vi "task.vi"() -> ()   [LabVIEW 2016, in "DGUS.lvlib"]
uses:
  DGUS.lvlib
  Control/state.ctl
  Control/data.ctl
  DGUS.lvclass
  <vilib>/Instr/_visa.llb/VISA Configure Serial Port (Instr).vi
panel:
  in  "停止":bool
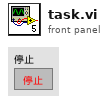
[diagram p1: front panel]
types:
  T1 = typedef "DGUS.lvlib/state.ctl" = enum16{"init", "open", "get data", "write buffer", "read buffer", "exit"}
  T2 = typedef "DGUS.lvlib/data.ctl" = cluster{"DGUS.lvclass":refnum<class "DGUS.lvclass">, "msgQueen":refnum<queue>, "VISA resource name":refnum<visa-resource-name>, "WriteBuffer":string, "ReadBuffer":string}
  T3 = cluster{"站点名称":string, "中文名称":string, "英文名称":string, "检测值":sgl, "小数位":u8, "单位":string, "页面":u16}[]
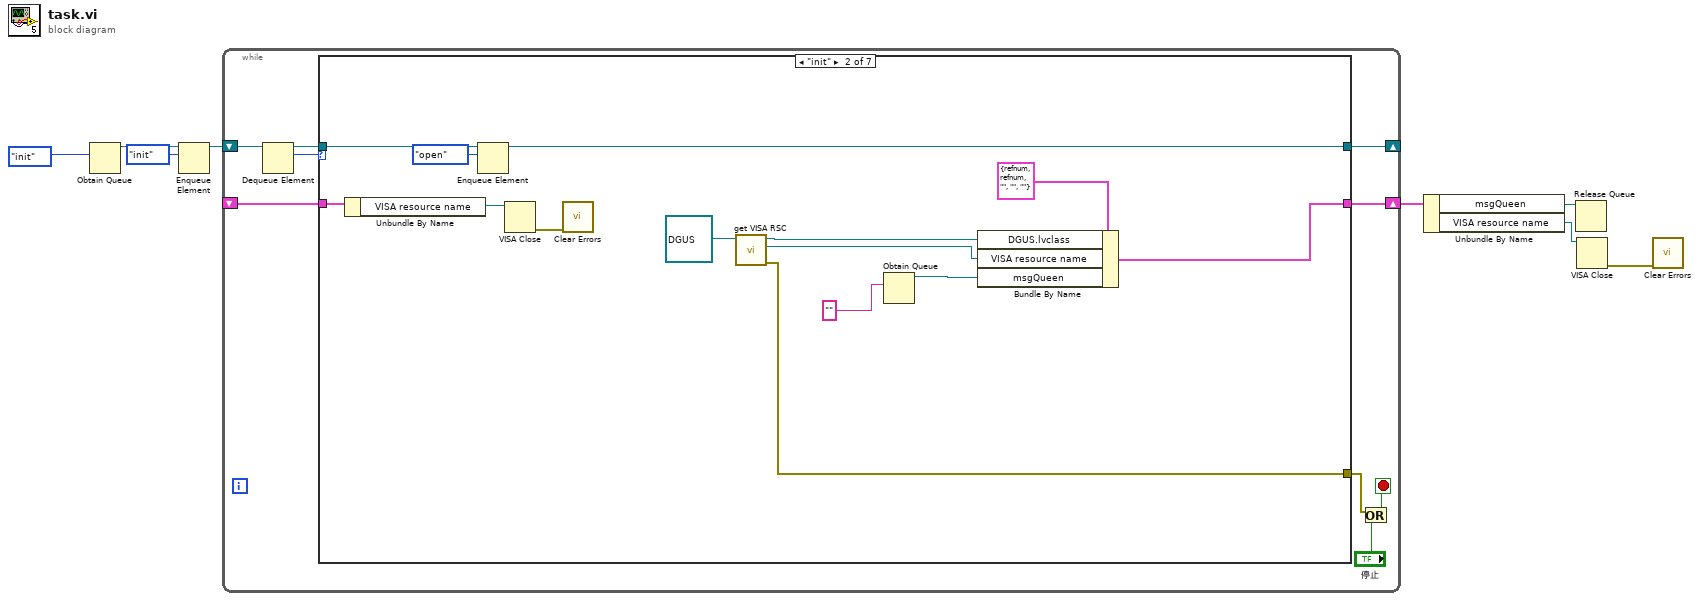
[diagram p0: block diagram]
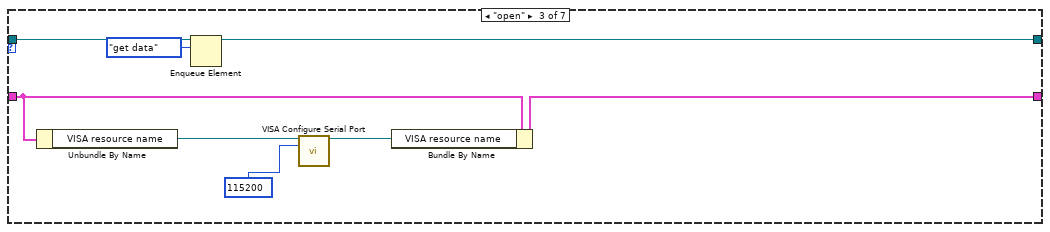
[diagram p3: hidden frame]
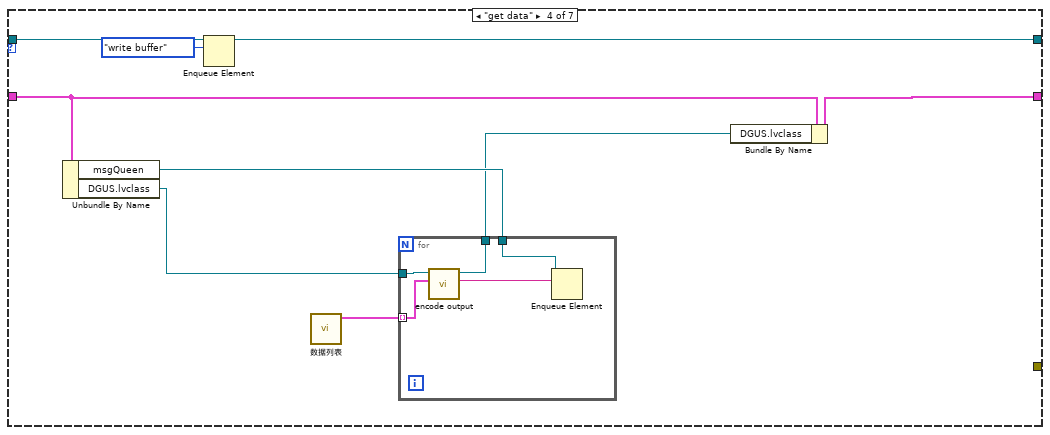
[diagram p4: hidden frame]
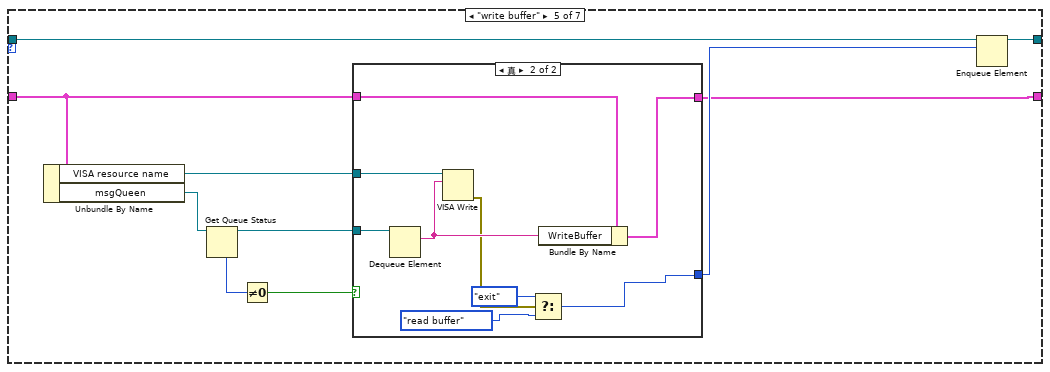
[diagram p5: hidden frame]
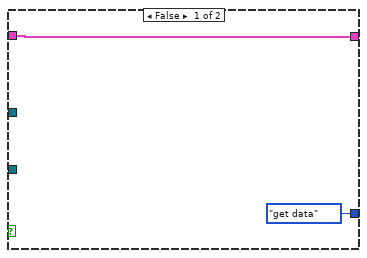
[diagram p6: hidden frame]
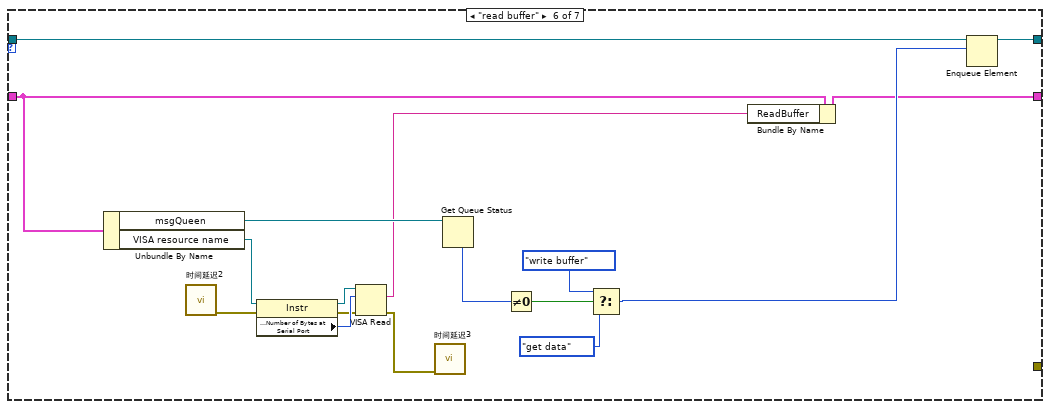
[diagram p7: hidden frame]
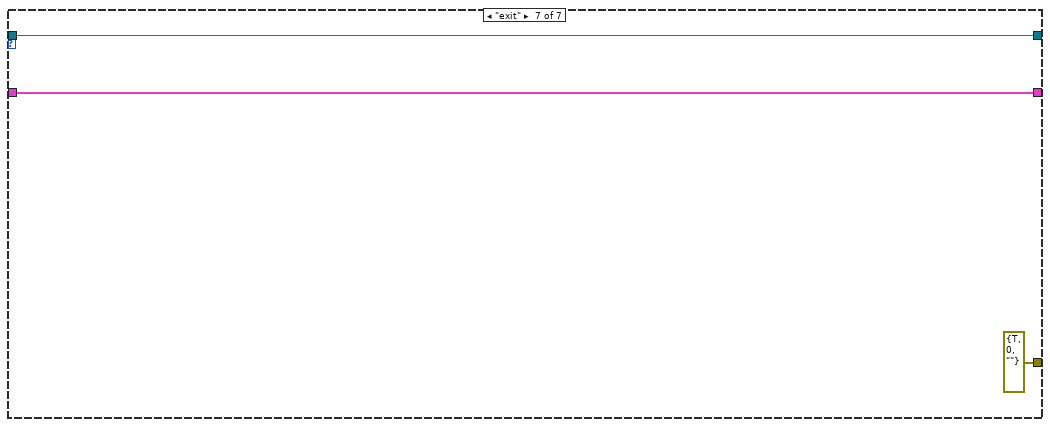
[diagram p8: hidden frame]
diagram:
  n1 = Obtain Queue(element data type=state."init" ("枚举")) -> (queue out=w7:refnum<queue>)  [unwired: 4 in, 2 out]
  n2 = Enqueue Element(queue=w7, element=state."init" ("元素")) -> (queue out=w6:refnum<queue>)  [unwired: 2 in, 2 out]
  n3 = while {
    shift-right: [w14] -> _
    shift-left: w6 -> [w17]
    shift-right: [w12] -> w4
    shift-left: _ -> [w13]
    stop <- w10 stop-if-true
    n4 = Dequeue Element(queue=w17) -> (queue out=w15:refnum<queue>, element=w16:T1)  [unwired: 2 in, 2 out]
    n5 = case shown="\"init\"" w16 {
      tunnel: w15 -> [w19 w33 w40 w50 w65 w93 w96]
      tunnel: [w19 w32 w39 w49 w62 w83 w96] -> w14
      tunnel: w13 -> [w18 w26 w38 w46 w57 w92 w95]
      tunnel: [w18 w30 w36 w45 w56 w81 w95] -> w12
      tunnel: [_ w20 _ _ _ _ errorcluster {"status"=TRUE, "code"=0, "source"=""} ("error out")] -> w9
      frame Default {
      }
      frame "init" {
        n6 = Unbundle By Name(w26) -> ("VISA resource name"=w25:refnum<visa-resource-name>)
        n7 = Enqueue Element(queue=w33, element=state."open" ("元素")) -> (queue out=w32:refnum<queue>)  [unwired: 2 in, 2 out]
        n8 = VISA Close(VISA resource name=w25) -> (error out=w24:errorcluster)  [unwired: 1 in]
        n9 = call <vilib>:"Clear Errors.vi"("error in (no error)"=w24) -> ()  [unwired: 5 in, 2 out]
        n10 = call "get VISA RSC.vi"("DGUS 输入"=refnum<class "DGUS.lvclass"> refnum ("DGUS.lvclass")) -> ("error out"=w20:errorcluster, "VISA资源名称"=w21:refnum<visa-resource-name>, "DGUS 输出"=w22:refnum<class "DGUS.lvclass">)  [unwired: 8 in]
        n11 = Obtain Queue(element data type="") -> (queue out=w29:refnum<queue>)  [unwired: 4 in, 2 out]
        n12 = Bundle By Name(cluster=T2 {"DGUS.lvclass"=refnum, "msgQueen"=refnum, "VISA resource name"="", "WriteBuffer"="", "ReadBuffer"=""}, "DGUS.lvclass"=w22, "VISA resource name"=w21, "msgQueen"=w29) -> (w30:T2)
      }
      frame "open" {
        n13 = Unbundle By Name(w38) -> ("VISA resource name"=w37:refnum<visa-resource-name>)
        n14 = Enqueue Element(queue=w40, element=state."get data" ("元素")) -> (queue out=w39:refnum<queue>)  [unwired: 2 in, 2 out]
        n15 = call-poly "VISA Configure Serial Port"("VISA resource name"=w37, "baud rate (9600)"=u32 115200) -> ("VISA resource name out"=w35:refnum<visa-resource-name>)  [unwired: 12 in, 1 out]
        n16 = Bundle By Name(cluster=w38, "VISA resource name"=w35) -> (w36:T2)
      }
      frame "get data" {
        n17 = Unbundle By Name(w46) -> ("msgQueen"=w47:refnum<queue>, "DGUS.lvclass"=w48:refnum<class "DGUS.lvclass">)
        n18 = Enqueue Element(queue=w50, element=state."write buffer" ("元素")) -> (queue out=w49:refnum<queue>)  [unwired: 2 in, 2 out]
        n19 = call "数据列表.vi"() -> ("数组"=w42:T3)  [unwired: 11 in]
        n20 = for {
          tunnel: w48 -> [w55]
          tunnel: w47 -> [w54]
          tunnel: [w52] -> w44
          tunnel: w42 -> [w51] mode=indexing
          n21 = call "encode output.vi"("data"=w51, "DGUS输入"=w55) -> ("数据帧"=w53:string, "DGUS输出"=w52:refnum<class "DGUS.lvclass">)  [unwired: 8 in]
          n22 = Enqueue Element(queue=w54, element=w53) -> ()  [unwired: 2 in, 3 out]
        }
        n23 = Bundle By Name(cluster=w46, "DGUS.lvclass"=w44) -> (w45:T2)
      }
      frame "write buffer" {
        n24 = Unbundle By Name(w57) -> ("VISA resource name"=w64:refnum<visa-resource-name>, "msgQueen"=w63:refnum<queue>)
        n25 = Get Queue Status(queue=w63) -> (queue out=w61:refnum<queue>, # elements in queue=w60:i32)  [unwired: 2 in, 6 out]
        n26 = Not Equal To 0?(x=w60) -> (x != 0?=w59:bool)
        n27 = case shown="真" w59 {
          tunnel: w64 -> [_ w76]
          tunnel: w61 -> [_ w75]
          tunnel: [state."get data" ("枚举") w69] -> w58
          tunnel: w57 -> [w67 w74]
          tunnel: [w67 w72] -> w56
          frame False {
          }
          frame True {
            n28 = Dequeue Element(queue=w75) -> (element=w73:string)  [unwired: 2 in, 3 out]
            n29 = VISA Write(VISA resource name=w76, write buffer=w73) -> (error out=w71:errorcluster)  [unwired: 1 in, 2 out]
            n30 = Select(t=state."exit", s=w71, f=state."read buffer" ("枚举")) -> (s? t:f=w69:T1)
            n31 = Bundle By Name(cluster=w74, "WriteBuffer"=w73) -> (w72:T2)
          }
        }
        n32 = Enqueue Element(queue=w65, element=w58) -> (queue out=w62:refnum<queue>)  [unwired: 2 in, 2 out]
      }
      frame "read buffer" {
        n33 = Unbundle By Name(w92) -> ("msgQueen"=w86:refnum<queue>, "VISA resource name"=w90:refnum<visa-resource-name>)
        n34 = call "时间延迟2"() -> ("error out"=w91:errorcluster)  [unwired: 11 in]
        n35 = property class="Instr"(reference=w90, error in=w91) -> (reference out=w89:refnum<visa-resource-name>, error out=w87:errorcluster, "Serial Settings:Number of Bytes at Serial Port"=w88:u32)
        n36 = VISA Read(VISA resource name=w89, byte count=w88, error in (no error)=w87) -> (read buffer=w80:string, error out=w77:errorcluster)  [unwired: 2 out]
        n37 = call "时间延迟3"("error in (no error)"=w77) -> ()  [unwired: 10 in, 1 out]
        n38 = Get Queue Status(queue=w86) -> (# elements in queue=w85:i32)  [unwired: 2 in, 7 out]
        n39 = Not Equal To 0?(x=w85) -> (x != 0?=w84:bool)
        n40 = Select(t=state."write buffer" ("枚举"), s=w84, f=state."get data" ("枚举")) -> (s? t:f=w82:T1)
        n41 = Bundle By Name(cluster=w92, "ReadBuffer"=w80) -> (w81:T2)
        n42 = Enqueue Element(queue=w93, element=w82) -> (queue out=w83:refnum<queue>)  [unwired: 2 in, 2 out]
      }
      frame "exit" {
      }
    }
    n43 = Or(x=w9, y="停止") -> (x .or. y?=w10:bool)
  }
  n44 = Unbundle By Name(w4) -> ("msgQueen"=w3:refnum<queue>, "VISA resource name"=w2:refnum<visa-resource-name>)
  n45 = Release Queue(queue=w3) -> ()  [unwired: 2 in, 3 out]
  n46 = VISA Close(VISA resource name=w2) -> (error out=w1:errorcluster)  [unwired: 1 in]
  n47 = call <vilib>:"Clear Errors.vi"("error in (no error)"=w1) -> ()  [unwired: 5 in, 2 out]
